vi "AFM_Litho_Plugin.IV.TestLauncher.vi"() -> ()   [LabVIEW 2019, in "AFM_Litho_Plugin.IV.lvclass"]
uses:
  AFM_Litho_Plugin.IV.lvclass
  <vilib>/JKI/JKI SMO/SMO/Typedefs/SMOState --Enum.ctl
  Typedefs/PrivateEvents--AFM_Litho_Plugin.IV.IV Run--Local.ctl
  C:/Program Files (x86)/National Instruments/LabVIEW 2019/vi.lib/JKI/JKI SMO/SMO/SMO.lvclass
  <vilib>/JKI/JKI SMO/SMO/SMO.lvclass/SMO.ctl
  AFM_Litho_Plugin.IV.lvclass/AFM_Litho_Plugin.IV.ctl
  <userlib>/LevyLab/Instrument Framework/SMOs/RemoteControl/Typedefs/RC Com Type--enum.ctl
  b9372eaf-d79d-420f-ae4a-5723e45e53aa.vi
  21cc0d15-aa5c-4e02-9f98-410864ffd08d.vi
  2cee4e23-403c-4d2f-920d-9f09caed685e.vi
  9af032d4-89d2-4663-9556-aa01e6123ab8.vi
  e51c5ca0-d227-4b24-97f1-175e48e65030.vi
  <vilib>/JKI/JKI SMO/SMO/Private/ReftoDVR--SMO.vi
  b9372eaf-d79d-420f-ae4a-5723e45e53aa.vi/303a33a2-dbc0-401d-b58e-53f0a523a2a2.vi
  b9372eaf-d79d-420f-ae4a-5723e45e53aa.vi/4d87f6fd-d19c-4d82-9aec-8cbcd500ecd7.vi
  21cc0d15-aa5c-4e02-9f98-410864ffd08d.vi/303a33a2-dbc0-401d-b58e-53f0a523a2a2.vi
  21cc0d15-aa5c-4e02-9f98-410864ffd08d.vi/4d87f6fd-d19c-4d82-9aec-8cbcd500ecd7.vi
  2cee4e23-403c-4d2f-920d-9f09caed685e.vi/303a33a2-dbc0-401d-b58e-53f0a523a2a2.vi
  2cee4e23-403c-4d2f-920d-9f09caed685e.vi/4d87f6fd-d19c-4d82-9aec-8cbcd500ecd7.vi
  9af032d4-89d2-4663-9556-aa01e6123ab8.vi/a9304a9f-69c7-45ea-b89b-09982a2100b8.vi
  e51c5ca0-d227-4b24-97f1-175e48e65030.vi/303a33a2-dbc0-401d-b58e-53f0a523a2a2.vi
  e51c5ca0-d227-4b24-97f1-175e48e65030.vi/4d87f6fd-d19c-4d82-9aec-8cbcd500ecd7.vi
  <vilib>/Utility/Data Type/Get Type Information.vi
  <vilib>/JDP Science/JSONtext/JSON text to Variant.vi
  <vilib>/Utility/LVClass/Get LV Class Name.vi
  <vilib>/JDP Science/JSONtext/LVClass Serializer/JSONtext LVClass Serializer.lvclass
  <vilib>/JKI/JKI SMO/SMO/SMO.lvclass
  <userlib>/LevyLab/Instrument Framework/SMOs/RemoteControl/RemoteControl.lvclass
panel:
  out "Start Status":string
  in  "IV Run Parameters":T1={"Pattern"=enum."Ramp /\\", "Cycles"=5.0, "Rate"=1.0, "End"=-1.0, "Start"=1.0}
  out "Help Reply":string[](array[string])
  out "ACK Reply":string
  in  "HELP":bool=TRUE
  in  "ACK":bool
  out "IV_ABORT Reply":string
  in  "IV_ABORT":bool
  out "IV_RUN Reply":string
  in  "IV_RUN":bool
  out "IV_Status Reply":string
  in  "IV_STATUS":bool=TRUE
  out "SMO State":T2
  out "error out":errorcluster
  in  "Stop":bool
  # "Measurement SMO Test Launcher"
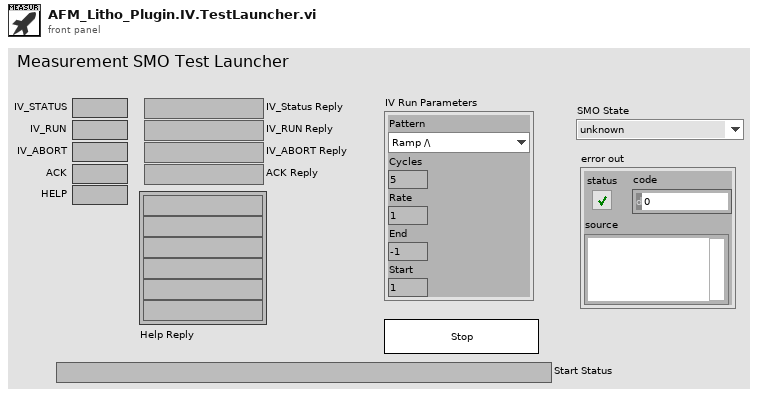
[diagram p1: front panel]
types:
  T1 = typedef "AFM_Litho_Plugin.IV.lvclass/PrivateEvents--AFM_Litho_Plugin.IV.IV Run--Local.ctl" = cluster{"Pattern":enum16{"Ramp /", "Ramp /\\", "Smooth Ramp _/", "Smooth Ramp _/\\_", "Frequency"}, "Cycles":dbl, "Rate":dbl, "End":dbl, "Start":dbl}
  T2 = typedef "SMO.lvclass/SMOState --Enum.ctl" = enum16{"unknown", "Created", "Started", "Stopped"}
  T3 = typedef "SMO.lvclass/Public Events.ctl" = cluster{"Error":refnum<user-event>, "State":refnum<user-event>, "Reserve State":refnum<user-event>}
  T4 = typedef "AFM_Litho_Plugin.IV.lvclass/PublicEvents--Cluster.ctl" = cluster{"StartStatus":refnum<user-event>}
  T5 = cluster{"Event Registration Refnum":refnum<event-registration>}
  T6 = typedef "RemoteControl.lvclass/RC Com Type--enum.ctl" = enum16{"RC", "STM", "ZMQ"}
  T7 = typedef "AFM_Litho_Plugin.IV.lvclass/PublicEvents--MeasurementSMO.StartStatus.ctl" = string
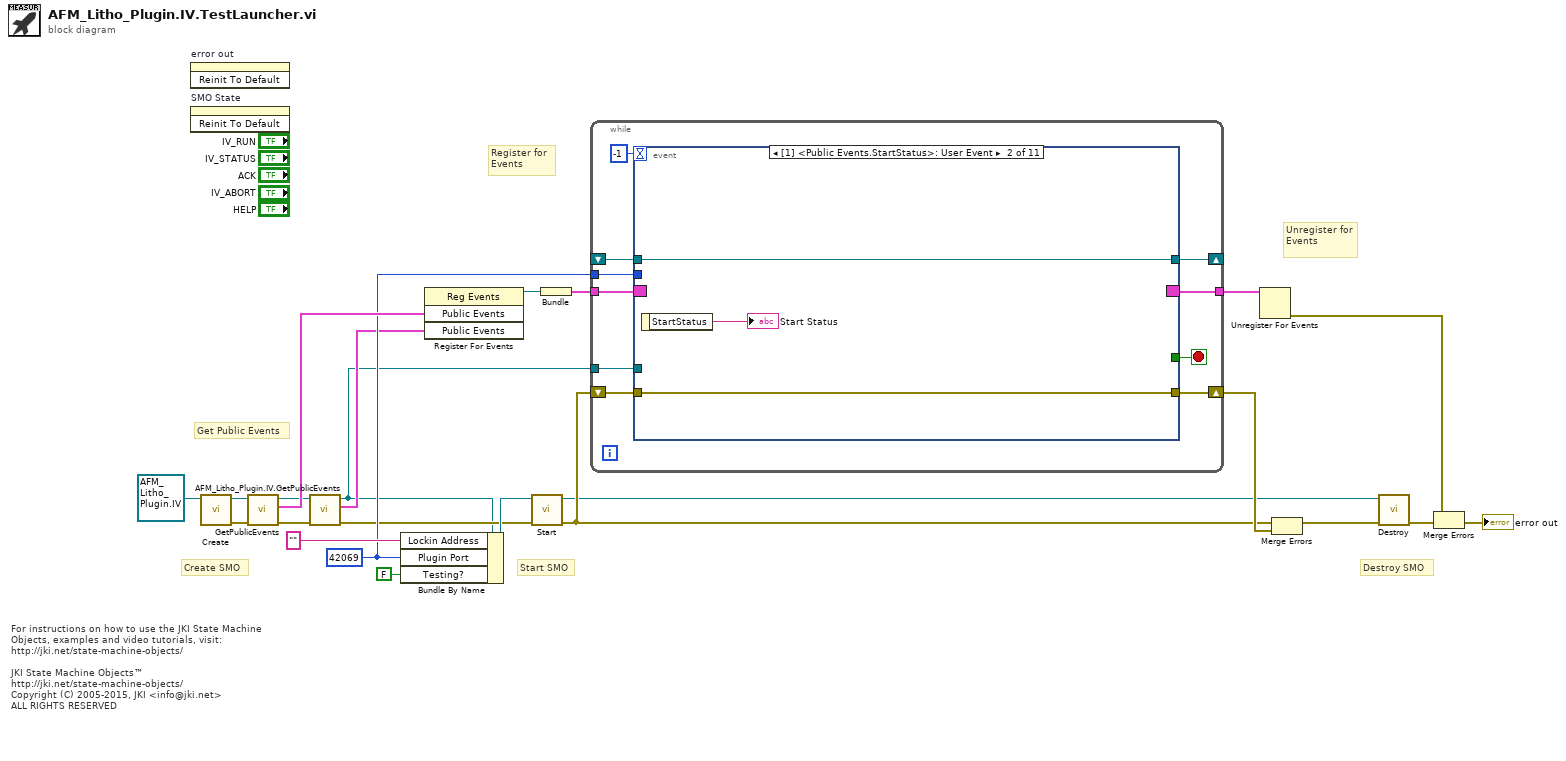
[diagram p0: block diagram]
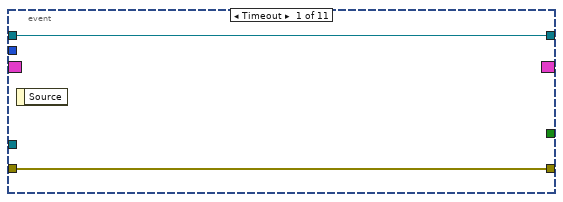
[diagram p2: hidden frame]
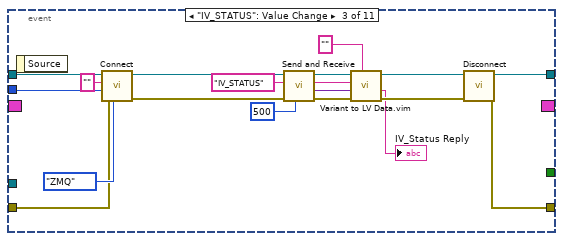
[diagram p3: hidden frame]
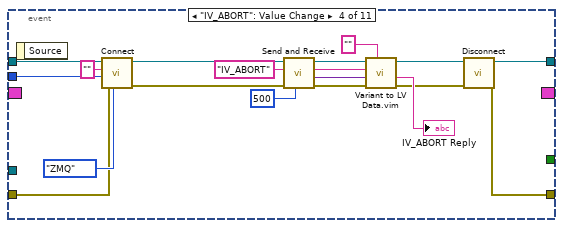
[diagram p4: hidden frame]
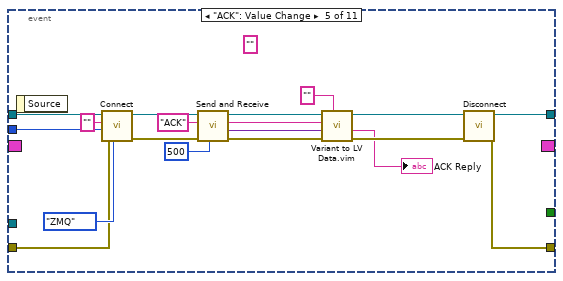
[diagram p5: hidden frame]
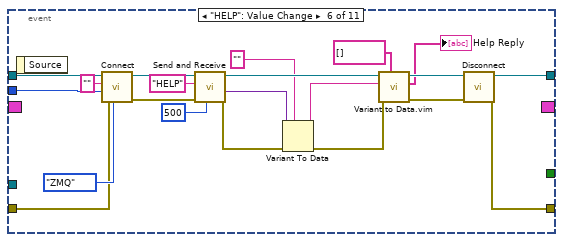
[diagram p6: hidden frame]
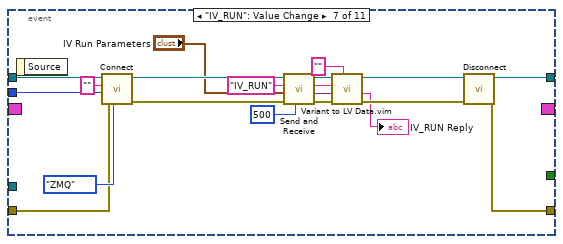
[diagram p7: hidden frame]
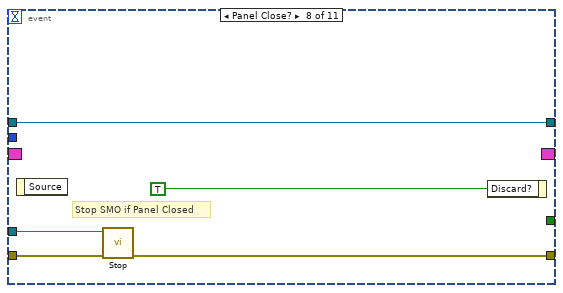
[diagram p8: hidden frame]
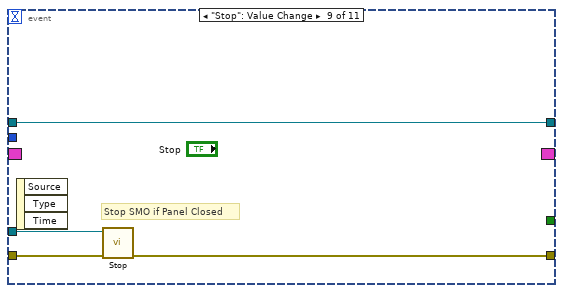
[diagram p9: hidden frame]
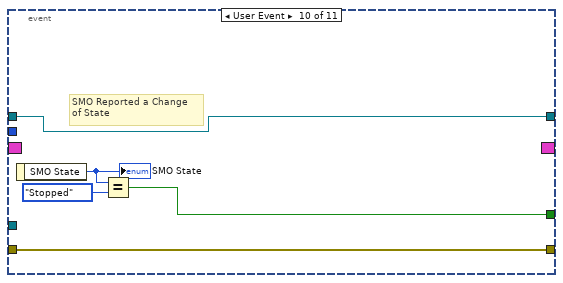
[diagram p10: hidden frame]
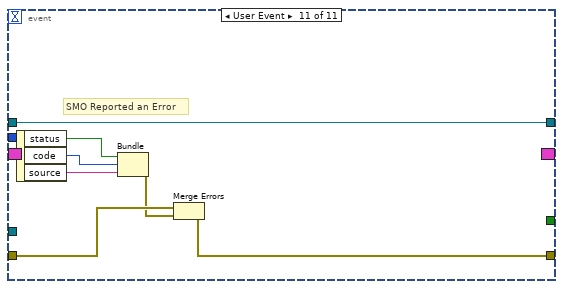
[diagram p11: hidden frame]
diagram:
  w7 = u16 42069 ("Plugin Port")
  # "For instructions on how to use the JKI State Machine Objects, examples and video tutorials, visit:\nhttp://jki.net/state-machine-objects/\n\nJKI State Machine Objects™\nhttp://jki.net/state-machine-objects/\nCopyright (C) 2005-2015, JKI <info@jki.net>\nALL RIGHTS RESERVED"
  # "Get Public Events"
  # "Start SMO"
  # "Destroy SMO"
  # "Create SMO"
  # "Unregister for Events"
  # "Register for Events"
  n1 = invoke on="error out" class="Clust (strict)" method="Reinit To Default"() -> ()  [unwired: 3 in, 3 out]
  n2 = invoke on="SMO State" class="Enum (strict)" method="Reinit To Default"() -> ()  [unwired: 3 in, 3 out]
  n3 = call <vilib>:"Create.vi"("SMO"=refnum<class "AFM_Litho_Plugin.IV.lvclass"> refnum ("SMO.Template.lvclass")) -> ("error out"=w12:errorcluster, "SMO out"=w13:refnum<class "AFM_Litho_Plugin.IV.lvclass">)  [unwired: 8 in, 1 out]
  n4 = call <vilib>:"GetPublicEvents.vi"("error in (no error)"=w12, "SMO"=w13) -> ("error out"=w5:errorcluster, "Public Events"=w11:T3, "SMO out"=w2:refnum<class "AFM_Litho_Plugin.IV.lvclass">)  [unwired: 7 in]
  n5 = call "AFM_Litho_Plugin.IV.GetPublicEvents.vi"("error in (no error)"=w5, "MeasurementSMO"=w2) -> ("error out"=w4:errorcluster, "Public Events"=w3:T4, "MeasurementSMO out"=w1:refnum<class "AFM_Litho_Plugin.IV.lvclass">)  [unwired: 7 in]
  n6 = Bundle By Name(cluster=w1, "Lockin Address"="" ("address"), "Plugin Port"=w7, "Testing?"=FALSE) -> (w9:refnum<class "AFM_Litho_Plugin.IV.lvclass">)
  n7 = register-events(w11, w3) -> (reference out=w10:refnum<event-registration>)  [unwired: 2 in, 1 out]
  n8 = call <vilib>:"Start.vi"("error in (no error)"=w4, "SMO"=w9) -> ("error out"=w16:errorcluster, "SMO out"=w14:refnum<class "AFM_Litho_Plugin.IV.lvclass">)  [unwired: 8 in]
  n9 = Bundle("Event Registration Refnum"=w10) -> (w22:T5)  [unwired: 1 in]
  n10 = while {
    shift-right: [w32] -> w21
    shift-left: w16 -> [w31]
    tunnel: w22 -> [w30]
    tunnel: [w29] -> w23
    tunnel: w1 -> [w28]
    shift-right: [w26] -> _
    shift-left: _ -> [w25]
    tunnel: w7 -> [w24]
    stop <- w33 stop-if-true
    n11 = event shown="[1] <Public Events.StartStatus>: User Event" {
      selector: w30 -> [_ _ _ _ _ _ _ _ _ _ _]
      dyn-events: [_ _ _ _ _ _ _ _ _ _ _] -> w29
      timeout: -1 -> [_ _ _ _ _ _ _ _ _ _ _]
      tunnel: [_ _ _ _ _ _ _ _ _ w143 _] -> w33
      tunnel: w28 -> [_ _ _ _ _ _ _ w137 w141 _ _]
      tunnel: [w35 w38 w51 w69 w88 w109 w127 w136 w140 w146 w151] -> w32
      tunnel: w31 -> [w35 w38 w50 w68 w87 w108 w126 w135 w139 w146 w149]
      tunnel: [w34 w37 w47 w65 w84 w105 w123 w133 w138 w142 w147] -> w26
      tunnel: w25 -> [w34 w37 w46 w64 w83 w104 w122 w133 w138 w142 w147]
      tunnel: w24 -> [_ _ w39 w57 w75 w93 w114 _ _ _ _]
      event Timeout {
        n12 = event-data() -> ()  [unwired: 1 in, 1 out]
      }
      event User Event {
        n13 = event-data() -> ("StartStatus"=→"Start Status":T7)  [unwired: 1 in]
      }
      event "IV_STATUS": Value Change {
        n14 = event-data() -> ()  [unwired: 1 in, 1 out]
        n15 = call <userlib>:"Connect.vi"("RC Type"=RC_Com_Type--enum."ZMQ", "error in (no error)"=w50, "Port"=w39, "address"="", "RemoteControl in"=w46) -> ("error out"=w52:errorcluster, "RemoteControl out"=w56:refnum<class "RemoteControl.lvclass">)  [unwired: 5 in]
        n16 = call <userlib>:"Send and Receive.vi"("timeout (ms) [500]"=500, "error in (no error)"=w52, "Command"="IV_STATUS", "RemoteControl in"=w56) -> ("error out"=w45:errorcluster, "Data out"=w41:variant, "Command out"=w42:string, "RemoteControl out"=w55:refnum<class "RemoteControl.lvclass">)  [unwired: 4 in]
        n17 = call "Variant to LV Data.vim"("type"="", "error in (no error)"=w45, "JSON Data in"=w41, "Command"=w42) -> ("error out"=w44:errorcluster, "Data out"=→"IV_Status Reply":string)  [unwired: 4 in, 2 out]
        n18 = call <userlib>:"Disconnect.vi"("error in (no error)"=w44, "RemoteControl in"=w55) -> ("error out"=w51:errorcluster, "RemoteControl out"=w47:refnum<class "RemoteControl.lvclass">)  [unwired: 8 in]
      }
      event "IV_ABORT": Value Change {
        n19 = event-data() -> ()  [unwired: 1 in, 1 out]
        n20 = call <userlib>:"Connect.vi"("RC Type"=RC_Com_Type--enum."ZMQ", "error in (no error)"=w68, "Port"=w57, "address"="", "RemoteControl in"=w64) -> ("error out"=w70:errorcluster, "RemoteControl out"=w74:refnum<class "RemoteControl.lvclass">)  [unwired: 5 in]
        n21 = call <userlib>:"Send and Receive.vi"("timeout (ms) [500]"=500, "error in (no error)"=w70, "Command"="IV_ABORT", "RemoteControl in"=w74) -> ("error out"=w60:errorcluster, "Data out"=w63:variant, "Command out"=w62:string, "RemoteControl out"=w73:refnum<class "RemoteControl.lvclass">)  [unwired: 4 in]
        n22 = call "Variant to LV Data.vim"("type"="", "error in (no error)"=w60, "JSON Data in"=w63, "Command"=w62) -> ("error out"=w58:errorcluster, "Data out"=→"IV_ABORT Reply":string)  [unwired: 4 in, 2 out]
        n23 = call <userlib>:"Disconnect.vi"("error in (no error)"=w58, "RemoteControl in"=w73) -> ("error out"=w69:errorcluster, "RemoteControl out"=w65:refnum<class "RemoteControl.lvclass">)  [unwired: 8 in]
      }
      event "ACK": Value Change {
        (unwired) ""
        n24 = event-data() -> ()  [unwired: 1 in, 1 out]
        n25 = call <userlib>:"Connect.vi"("RC Type"=RC_Com_Type--enum."ZMQ", "error in (no error)"=w87, "Port"=w75, "address"="", "RemoteControl in"=w83) -> ("error out"=w89:errorcluster, "RemoteControl out"=w92:refnum<class "RemoteControl.lvclass">)  [unwired: 5 in]
        n26 = call <userlib>:"Send and Receive.vi"("timeout (ms) [500]"=500, "error in (no error)"=w89, "Command"="ACK", "RemoteControl in"=w92) -> ("error out"=w82:errorcluster, "Data out"=w80:variant, "Command out"=w79:string, "RemoteControl out"=w76:refnum<class "RemoteControl.lvclass">)  [unwired: 4 in]
        n27 = call "Variant to LV Data.vim"("type"="", "error in (no error)"=w82, "JSON Data in"=w80, "Command"=w79) -> ("error out"=w81:errorcluster, "Data out"=→"ACK Reply":string)  [unwired: 4 in, 2 out]
        n28 = call <userlib>:"Disconnect.vi"("error in (no error)"=w81, "RemoteControl in"=w76) -> ("error out"=w88:errorcluster, "RemoteControl out"=w84:refnum<class "RemoteControl.lvclass">)  [unwired: 8 in]
      }
      event "HELP": Value Change {
        n29 = event-data() -> ()  [unwired: 1 in, 1 out]
        n30 = call <userlib>:"Connect.vi"("RC Type"=RC_Com_Type--enum."ZMQ", "error in (no error)"=w108, "Port"=w93, "address"="", "RemoteControl in"=w104) -> ("error out"=w110:errorcluster, "RemoteControl out"=w113:refnum<class "RemoteControl.lvclass">)  [unwired: 5 in]
        n31 = call <userlib>:"Send and Receive.vi"("timeout (ms) [500]"=500, "error in (no error)"=w110, "Command"="HELP", "RemoteControl in"=w113) -> ("error out"=w98:errorcluster, "Data out"=w94:variant, "RemoteControl out"=w102:refnum<class "RemoteControl.lvclass">)  [unwired: 4 in, 1 out]
        n32 = Variant To Data(error in=w98, type="", Variant=w94) -> (data=w95:string, error out=w97:errorcluster)
        n33 = call "Variant to Data.vim"("Data Type"=string[] [], "error in (no error)"=w97, "Data in"=w95, "RemoteControl in"=w102) -> ("error out"=w96:errorcluster, "Data out"=→"Help Reply":string[], "RemoteControl out"=w103:refnum<class "RemoteControl.lvclass">)  [unwired: 5 in]
        n34 = call <userlib>:"Disconnect.vi"("error in (no error)"=w96, "RemoteControl in"=w103) -> ("error out"=w109:errorcluster, "RemoteControl out"=w105:refnum<class "RemoteControl.lvclass">)  [unwired: 8 in]
      }
      event "IV_RUN": Value Change {
        n35 = event-data() -> ()  [unwired: 1 in, 1 out]
        n36 = call <userlib>:"Connect.vi"("RC Type"=RC_Com_Type--enum."ZMQ", "error in (no error)"=w126, "Port"=w114, "address"="", "RemoteControl in"=w122) -> ("error out"=w128:errorcluster, "RemoteControl out"=w132:refnum<class "RemoteControl.lvclass">)  [unwired: 5 in]
        n37 = call <userlib>:"Send and Receive.vi"("timeout (ms) [500]"=500, "error in (no error)"=w128, "Data"="IV Run Parameters", "Command"="IV_RUN", "RemoteControl in"=w132) -> ("error out"=w120:errorcluster, "Data out"=w118:variant, "Command out"=w117:string, "RemoteControl out"=w131:refnum<class "RemoteControl.lvclass">)  [unwired: 3 in]
        n38 = call "Variant to LV Data.vim"("type"="", "error in (no error)"=w120, "JSON Data in"=w118, "Command"=w117) -> ("error out"=w119:errorcluster, "Data out"=→"IV_RUN Reply":string)  [unwired: 4 in, 2 out]
        n39 = call <userlib>:"Disconnect.vi"("error in (no error)"=w119, "RemoteControl in"=w131) -> ("error out"=w127:errorcluster, "RemoteControl out"=w123:refnum<class "RemoteControl.lvclass">)  [unwired: 8 in]
      }
      event Panel Close? {
        # "Stop SMO if Panel Closed"
        n40 = event-data() -> ()  [unwired: 1 in, 1 out]
        n41 = call <vilib>:"Stop.vi"("error in (no error)"=w135, "SMO"=w137) -> ("error out"=w136:errorcluster)  [unwired: 8 in, 1 out]
        n42 = event-data("Discard?"=TRUE ("OK")) -> ()  [unwired: 1 in, 1 out]
      }
      event "Stop": Value Change {
        # "Stop SMO if Panel Closed"
        n43 = event-data() -> ()  [unwired: 1 in, 3 out]
        n44 = call <vilib>:"Stop.vi"("error in (no error)"=w139, "SMO"=w141) -> ("error out"=w140:errorcluster)  [unwired: 8 in, 1 out]
      }
      event User Event {
        # "SMO Reported a Change\nof State"
        n45 = event-data() -> ("SMO State"=w145:T2)  [unwired: 1 in]
        "SMO State" <- w145
        n46 = Equal?(x=w145, y=SMOState_--Enum."Stopped") -> (x = y?=w143:bool)
      }
      event User Event {
        # "SMO Reported an Error"
        n47 = event-data() -> ("status"=w150:bool, "code"=w153:i32, "source"=w152:string)  [unwired: 1 in]
        n48 = Bundle("status"=w150, "code"=w153, "source"=w152) -> (w148:errorcluster)  [unwired: 1 in]
        n49 = Merge Errors(w149, w148) -> (w151:errorcluster)
      }
    }
  }
  n50 = Unregister For Events(event registration refnum=w23) -> (error out=w20:errorcluster)  [unwired: 1 in]
  n51 = Merge Errors(w16, w21) -> (w15:errorcluster)
  n52 = call <vilib>:"Destroy.vi"("error in (no error)"=w15, "SMO"=w14) -> ("error out"=w18:errorcluster)  [unwired: 9 in]
  n53 = Merge Errors(w20, w18) -> (→"error out":errorcluster)
